vi "SMSL-Drill FPGA.vi"() -> ()   [LabVIEW 2014]
uses:
  <vilib>/Platform/TimedLoop/XDataNode/timing_clust.ctl
  <vilib>/Platform/TimedLoop/XDataNode/nitl_modes.ctl
  <vilib>/Platform/TimedLoop/XDataNode/wakeup.ctl
  <vilib>/rvi/Emulation/niFpgaGetClockAttributes.vi
  <vilib>/rvi/Emulation/niFpgaSctlEmulationGetInTimedLoop.vi
  <vilib>/rvi/Emulation/niFpgaEmulationReportErrorSimple.vi
  <vilib>/rvi/eio/common/nirviEmuTemplateMethod_errors.vi
  <vilib>/rvi/Emulation/niFpgaCriticalErrorInLSC.vi
  <vilib>/eio/EIONode/EIONode.xnode
  <vilib>/Platform/TimedLoop/XDataNode/XDataNode.xnode
  <vilib>/Platform/TimedLoop/XDataNode/XDNodeRunTimeDep.lvlib
panel:
  out "Mod2/AI0":fxp<+/-,24,5>
  out "Bit Position":i32
  in  "Direction BKWD":bool
  in  "Direction FWD":bool
  in  "Enable/Disable":bool
  in  "frequency (periods/tick)":fxp<+,32,0>
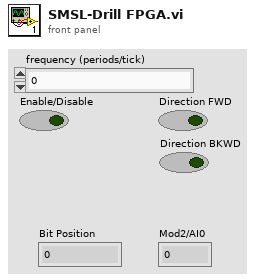
[diagram p1: front panel]
types:
  T1 = typedef "XDNodeRunTimeDep.lvlib/timing_clust.ctl" = cluster{"Expected End [f-1]":u64, "Actual End [f-1]":u64, "Finished Late? [f-1]":bool, "Expected End [i-1]":u64, "Actual End [i-1]":u64, "Finished Late? [i-1]":bool, "Expected Start [i]":u64, "Actual Start [i]":u64, "Expected Start [f]":u64, "Actual Start [f]":u64, "Source Name":string, "Structure Name":string, "Period":i64, "Deadline":i64, "Offset":i64, "Start":i64, "Priority":i32, "Timeout":i32, "Mode":T2, "Wakeup Reason":T3, "Error":errorcluster, "Source Type":string, "Secondary Source Type":string, "Global End Time":u64, "Global Start Time":u64, "Frame Duration":u64, "Iteration Duration":u64, "Assigned CPU":i32, "I/O Scan Engine Mode":u32}
  T2 = typedef "XDNodeRunTimeDep.lvlib/nitl_modes.ctl" = enum32{"No Change", "Process missed periods, maintain original phase", "Discard missed periods, maintain original phase", "Process missed periods, ignore original phase", "Discard missed periods, ignore original phase"}
  T3 = typedef "XDNodeRunTimeDep.lvlib/wakeup.ctl" = enum32{"Normal", "Aborted", "Asynchronous wakeup", "Timing source error", "Timed loop error", "Timeout"}
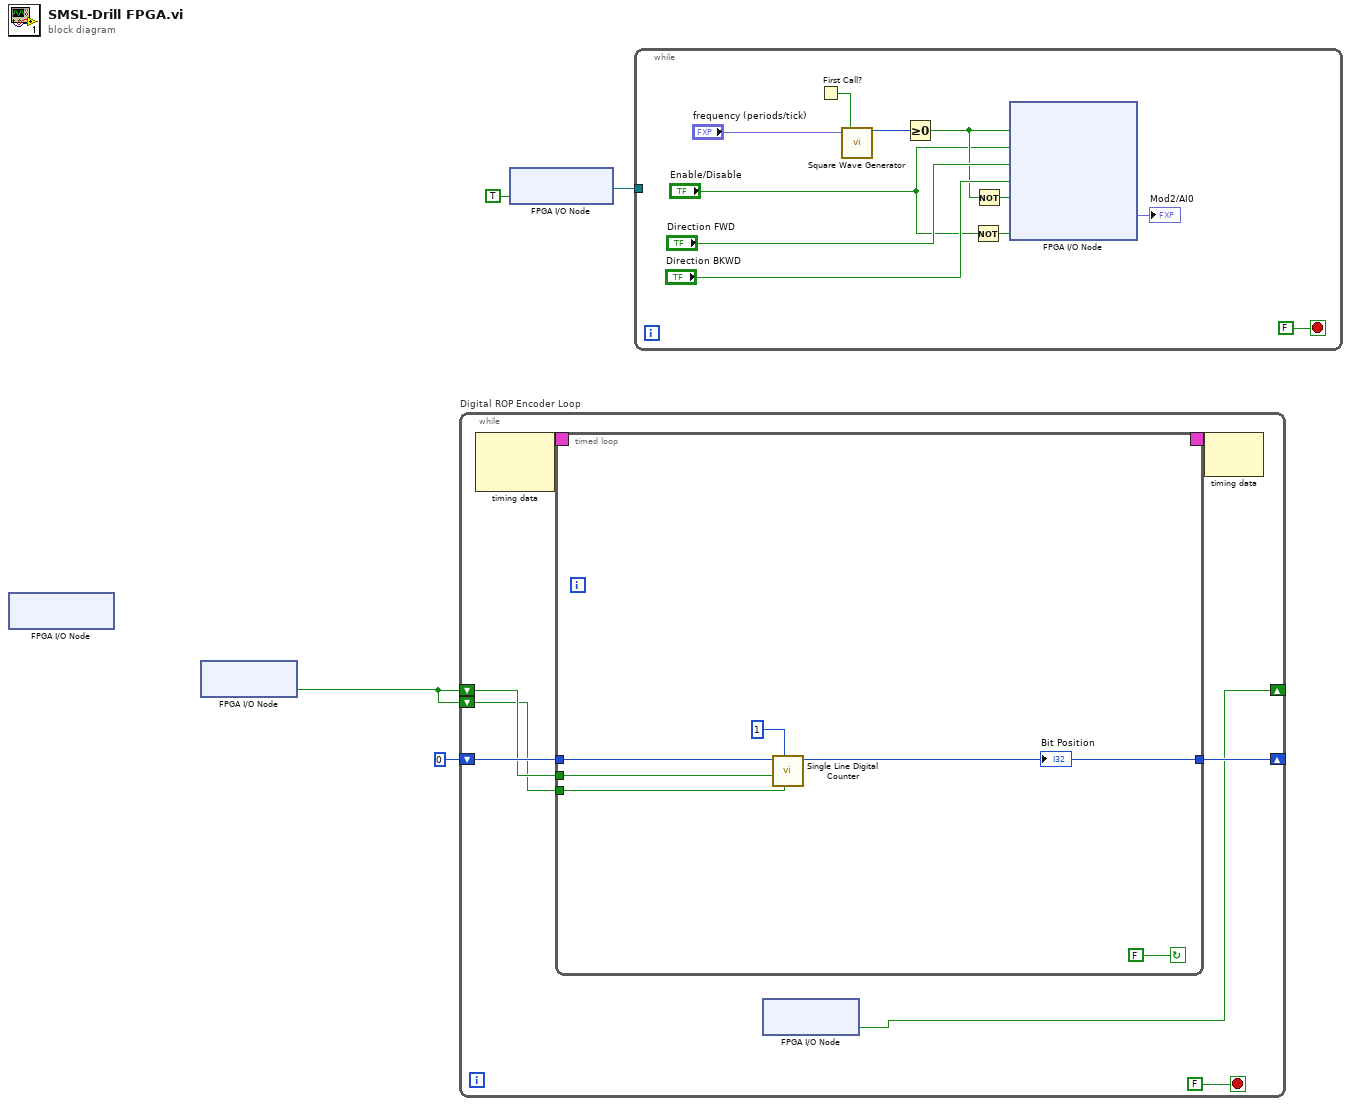
[diagram p0: block diagram]
diagram:
  n1 = xnode "FPGA I/O Node"() -> ()  [unwired: 1 in, 2 out]
  n2 = xnode "FPGA I/O Node"() -> ("Mod3/DI0"=w3:bool)  [unwired: 1 in, 1 out]
  n3 = while "Digital ROP Encoder Loop" {
    shift-right: [w10] -> _
    shift-left: 0 ("New Count") -> [w11]
    shift-right: [w5] -> _
    shift-left: w3 -> [w9]
    shift-left: w3 -> [w6]
    stop <- FALSE stop-if-true
    n4 = node-c288 ("Input Node")() -> (w7:T1)  [unwired: 2 in]
    n5 = timed-loop "Timed Loop" {
      tunnel: w9 -> [w16]
      tunnel: w6 -> [w15]
      tunnel: [w14] -> w10
      tunnel: w11 -> [w18]
      timing-out: [_] -> w8
      timing: w7 -> [_]
      stop <- FALSE continue-if-true
      n6 = call "Single Line Digital Counter.vi"("Digital Line - Previous"=w15, "Counts per pulse"=1, "Digital Line"=w16, "Count In"=w18) -> ("Count Out"=w14:i32)  [unwired: 7 in]
      "Bit Position" <- w14
    }
    n7 = xnode "FPGA I/O Node"() -> ("Mod3/DI0"=w5:bool)  [unwired: 1 in, 1 out]
    n8 = node-c288(w8) -> ()  [unwired: 1 out]
  }
  n9 = xnode "FPGA I/O Node"("Mod2/Start"=TRUE) -> ("FPGA I/O Out"=w1:refnum<k21>)  [unwired: 1 in]
  n10 = while {
    tunnel: w1 -> [_]
    stop <- FALSE stop-if-true
    n11 = First Call?() -> (First Call?: T/F=w31:bool)
    n12 = call "Square Wave Generator"("frequency (periods/tick)"="frequency (periods/tick)", "reset"=w31) -> ("square wave out"=w30:i16)  [unwired: 13 in]
    n13 = Greater Or Equal To 0?(x=w30) -> (x >= 0?=w26:bool)
    n14 = Not(x="Enable/Disable") -> (.not. x?=w24:bool)
    n15 = Not(x=w26) -> (.not. x?=w27:bool)
    n16 = xnode "FPGA I/O Node"("Frequecy+"=w26, "Enable/Disable"="Enable/Disable", "Direction FWD"="Direction FWD", "Direction BKWD"="Direction BKWD", "Frequecy-"=w27, "Enable/Disable-"=w24) -> ("Mod2/AI0"=→"Mod2/AI0":fxp<+/-,24,5>)  [unwired: 7 in, 7 out]
  }
